vi "Demo_NIringData.vi"() -> ()   [LabVIEW 2021, in "RocketPlotDemo.lvlib"]
uses:
  Demo/RocketPlotDemo.lvlib
  TypeDefs/plot load data V2.ctl
  TypeDefs/plot properties V2.ctl
  TypeDefs/plot attributes V2.ctl
  TypeDefs/Plot scale axis properties.ctl
  TypeDefs/Plot general properties.ctl
  Classes/RocketPlotHandle/SubVIs/Init Options.ctl
  TypeDefs/TimeZone.ctl
  Classes/RocketPlotPanel/RocketPlotPanel.lvclass/RocketPlotPanel.ctl
  Demo/SubVIs/ring buffer data.ctl
  Classes/RocketPlotPanel/Read RocketPlotHandle.vi
  Classes/NIringPlotHandle/NIringPlotHandle.lvclass
  C:/Users/bjustice/Documents/GitHub/BluePlot/Source/Classes/RocketPlotHandle/RocketPlotHandle.lvclass
  Classes/RocketPlotPanel/RocketPlotPanel.lvclass
  C:/Program Files/National Instruments/LabVIEW 2021/vi.lib/IlluminatedG/IG OOPanel/OOPanel/Panel/Panel.lvclass
  Classes/RocketPlotHandle/Load PlotConfig.vi
  Classes/RocketPlotHandle/RocketPlotHandle.lvclass
  Classes/RocketPlotHandle/Get PlotConfig.vi
  <vilib>/National Instruments/Variant Ring Buffer/Ring Buffer.lvclass
  RocketPlot.lvlib
  <vilib>/IlluminatedG/IG OOPanel/OOPanel/Manager/Manager.lvclass
  C:/Users/bjustice/Documents/GitHub/BluePlot/Source/Classes/NIringPlotHandle/NIringPlotHandle.lvclass
  C:/Users/bjustice/Documents/GitHub/BluePlot/Source/Classes/RocketPlotPanel/RocketPlotPanel.lvclass
panel:
  in  "load config":bool
  in  "get config":bool
  out "time to plot":dbl
  out "Subscribed names":i32(listbox)
  in  "Plot config":T1={"plots"=[], "X-axis"={"Name Label.Text"="", "Style"=0, "Tick Colors:Minor Tick Color"=0, "Tick Colors:Tick Color"=0, "Marker Colors:Text Color"=0, "Grid Colors:Major Color"=0, "Grid Colors:Minor Color"=0, "Mapping Mode"=0, "Flipped"=FALSE, "Name Label.Visible"=FALSE, "Name Label.Text Colors:Text Color"=0, "Scale Fit"=0, "Range:Maximum"=0.0, "Range:Minimum"=0.0, "Offset and Multiplier:Multiplier"=0.0, "Offset and Multiplier:Offset"=0.0, "Name Label.Font:Size"=0, "Marker.Font:Size"=0, "Uniform Marker Spacing?"=TRUE, "Format String"=""}, "Y-axes"=[], "General"={"Title"="", "Time to Plot"=1800.0, "Title.Visible"=FALSE, "Sidebar.Visible"=FALSE, "Plot Area:Colors:BG Color"=0, "X Scale.Plot Name"="", "X Scale.Use Plot Name"=FALSE}} {"General"."Time to Plot" format="%<%M:%S>t"}
  # "Documentation and user guide:"
  # "https://github.com/justiceb/BluePlot/blob/main/README.md"
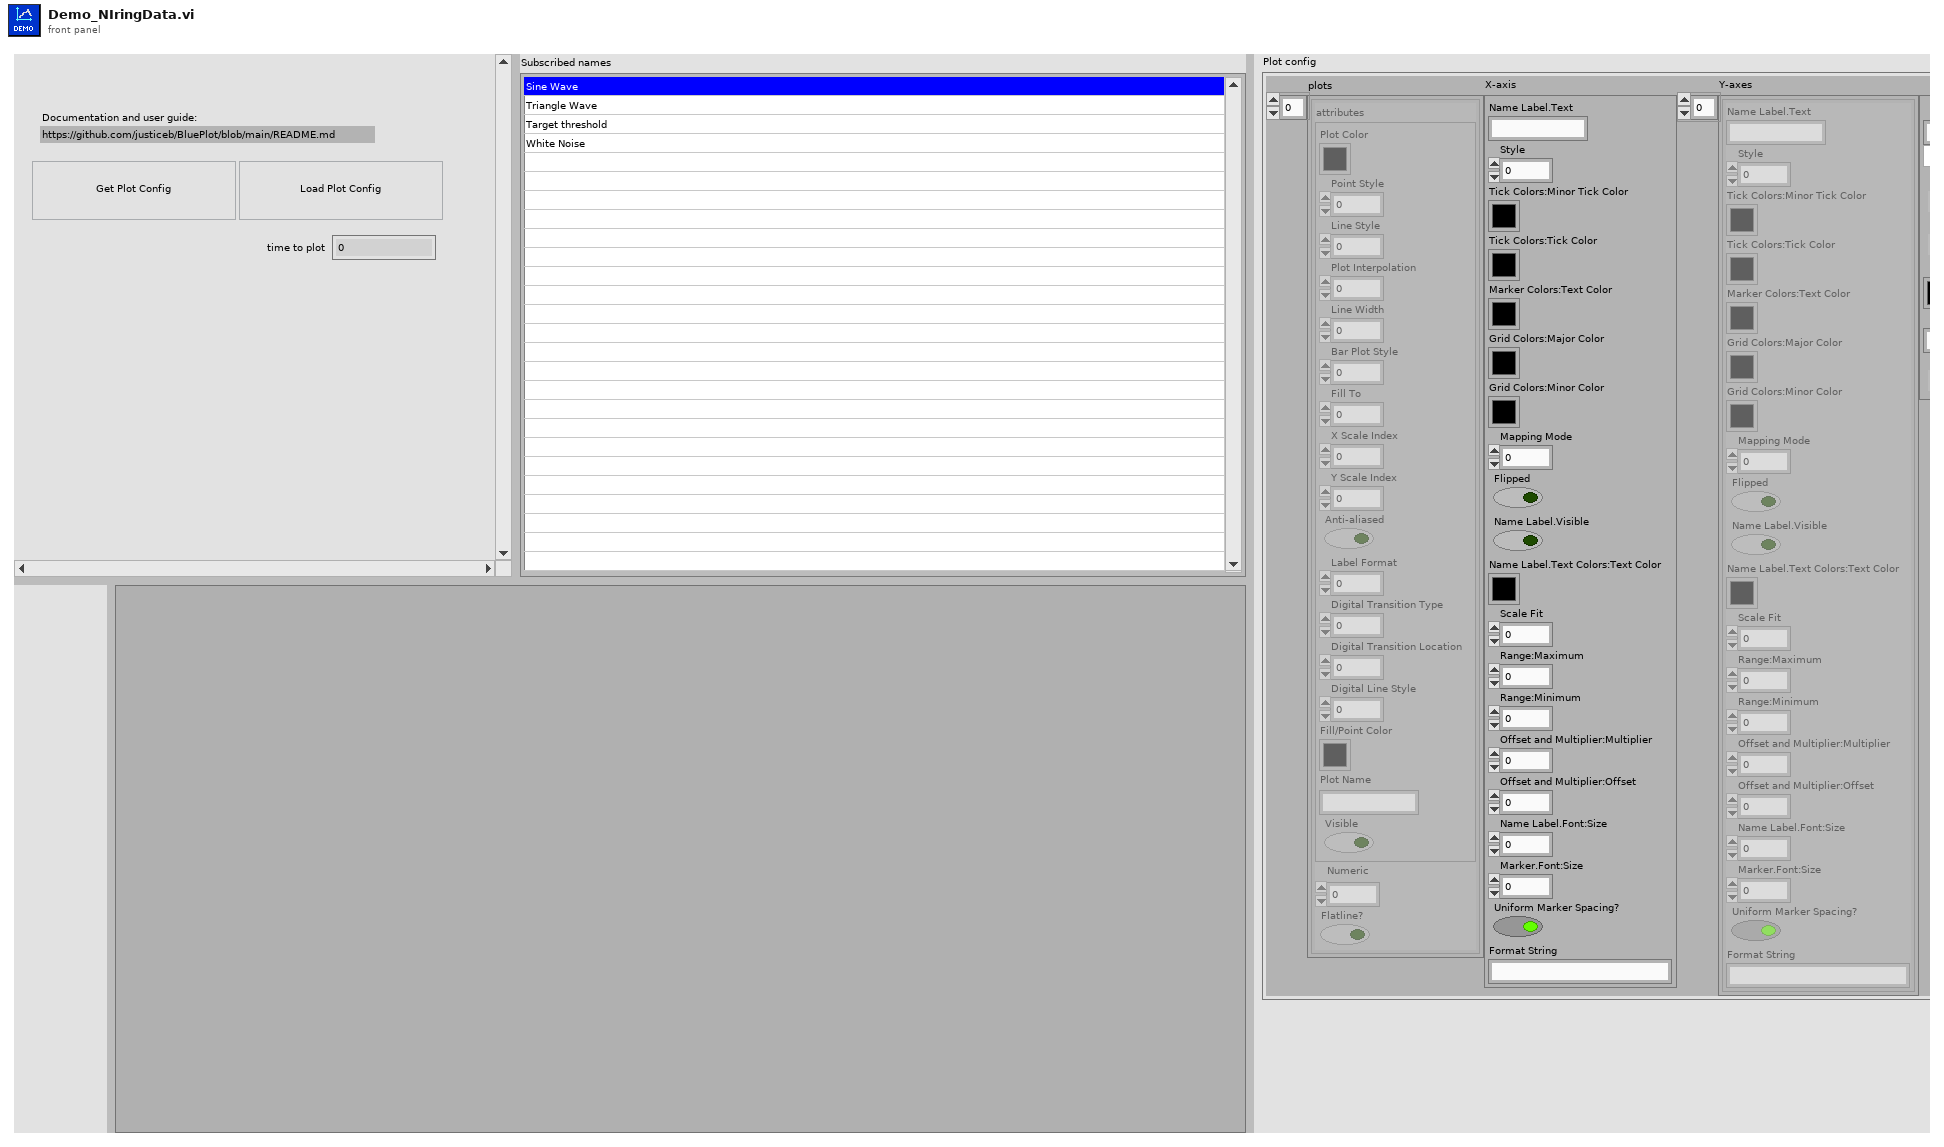
[diagram p1: front panel]
types:
  T1 = typedef "RocketPlot.lvlib/plot load data V2.ctl" = cluster{"plots":T2[], "X-axis":T4, "Y-axes":T4[], "General":T5}
  T2 = typedef "RocketPlot.lvlib/plot properties V2.ctl" = cluster{"attributes":T3, "Numeric":dbl, "Flatline?":bool}
  T3 = typedef "RocketPlot.lvlib/plot attributes V2.ctl" = cluster{"Plot Color":u32, "Point Style":u8, "Line Style":u8, "Plot Interpolation":u8, "Line Width":u8, "Bar Plot Style":u8, "Fill To":i16, "X Scale Index":u32, "Y Scale Index":u32, "Anti-aliased":bool, "Label Format":u8, "Digital Transition Type":u8, "Digital Transition Location":u8, "Digital Line Style":u8, "Fill/Point Color":u32, "Plot Name":string, "Visible":bool}
  T4 = typedef "RocketPlot.lvlib/Plot scale axis properties.ctl" = cluster{"Name Label.Text":string, "Style":u8, "Tick Colors:Minor Tick Color":u32, "Tick Colors:Tick Color":u32, "Marker Colors:Text Color":u32, "Grid Colors:Major Color":u32, "Grid Colors:Minor Color":u32, "Mapping Mode":u8, "Flipped":bool, "Name Label.Visible":bool, "Name Label.Text Colors:Text Color":u32, "Scale Fit":u8, "Range:Maximum":dbl, "Range:Minimum":dbl, "Offset and Multiplier:Multiplier":dbl, "Offset and Multiplier:Offset":dbl, "Name Label.Font:Size":u32, "Marker.Font:Size":u32, "Uniform Marker Spacing?":bool, "Format String":string}
  T5 = typedef "RocketPlot.lvlib/Plot general properties.ctl" = cluster{"Title":string, "Time to Plot":dbl, "Title.Visible":bool, "Sidebar.Visible":bool, "Plot Area:Colors:BG Color":u32, "X Scale.Plot Name":string, "X Scale.Use Plot Name":bool}
  T6 = typedef "RocketPlotHandle.lvclass/Init Options.ctl" = cluster{"UI visible?":bool, "Update rate (ms)":u32, "Sidebar.Visible":bool, "time to plot (init)":dbl, "time to plot (max)":dbl, "config file start path":path, "Title.Visible":bool, "Title":string, "TimeZone":T7}
  T7 = typedef "RocketPlot.lvlib/TimeZone.ctl" = enum16{"UTC", "Local"}
  T8 = typedef "RocketPlotDemo.lvlib/ring buffer data.ctl" = cluster{"timestamp":dbl, "value":dbl}
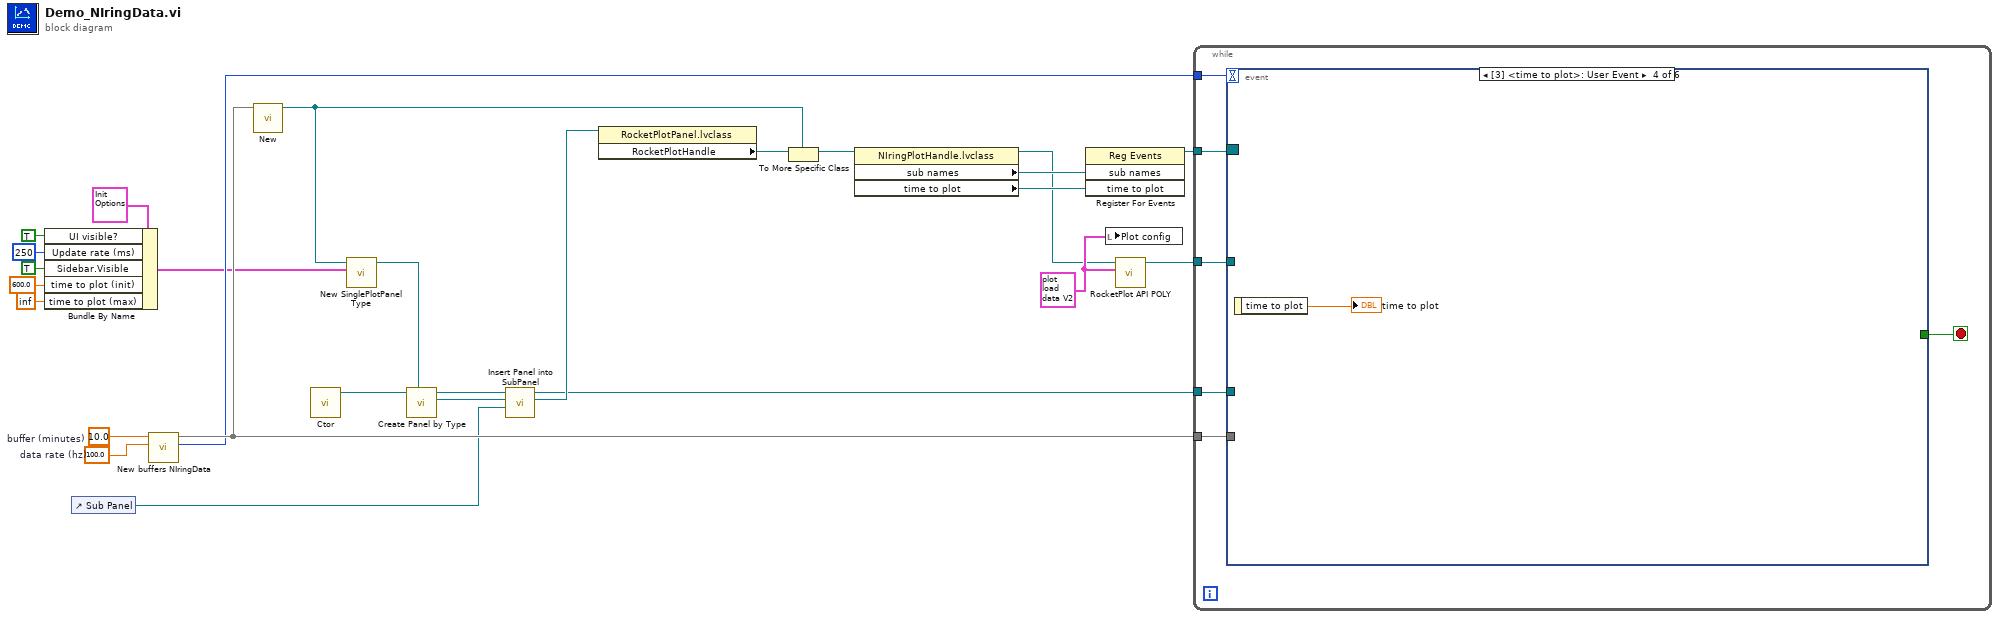
[diagram p0: block diagram]
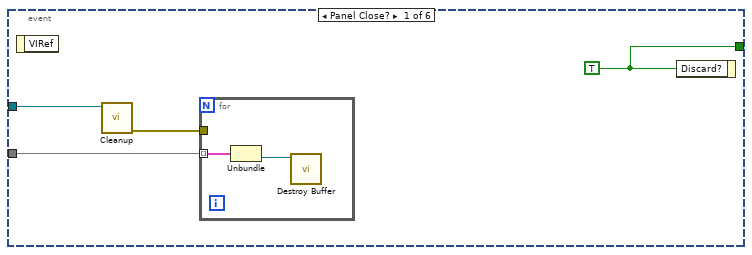
[diagram p2: hidden frame]
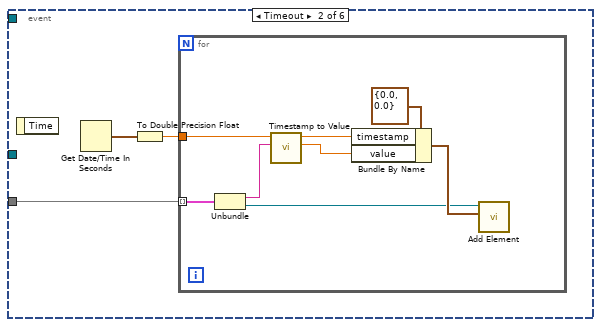
[diagram p3: hidden frame]
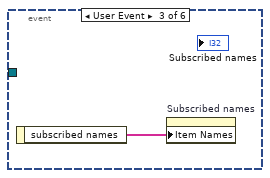
[diagram p4: hidden frame]
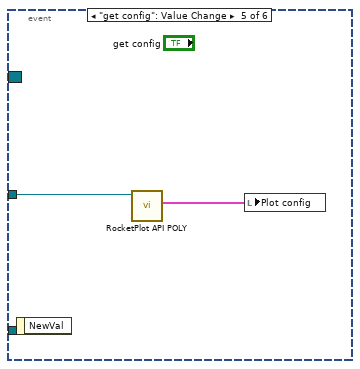
[diagram p5: hidden frame]
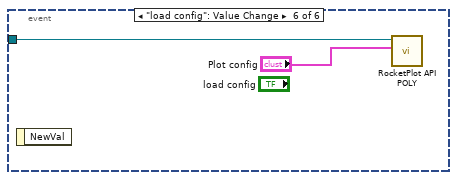
[diagram p6: hidden frame]
diagram:
  w21 = T1 {"plots"=[{"attributes"={"Plot Color"=16711680, "Point Style"=0, "Line Style"=0, "Plot Interpolation"=2, "Line Width"=0, "Bar Plot Style"=0, "Fill To"=-1, "X Scale Index"=0, "Y Scale Index"=0, "Anti-aliased"=FALSE, "Label Format"=3, "Digital Transition Type"=0, "Digital Transition Location"=2, "Digital Line Style"=1, "Fill/Point Color"=16711680, "Plot Name"="Sine Wave", "Visible"=TRUE}, "Numeric"=0.0, "Flatline?"=FALSE}, {"attributes"={"Plot Color"=4387583, "Point Style"=0, "Line Style"=0, "Plot Interpolation"=2, "Line Width"=0, "Bar Plot Style"=0, "Fill To"=-1, "X Scale Index"=0, "Y Scale Index"=1, "Anti-aliased"=FALSE, "Label Format"=3, "Digital Transition Type"=0, "Digital Transition Location"=2, "Digital Line Style"=1, "Fill/Point Color"=4387583, "Plot Name"="Triangle Wave", "Visible"=TRUE}, "Numeric"=0.0, "Flatline?"=FALSE}, {"attributes"={"Plot Color"=16722671, "Point Style"=0, "Line Style"=0, "Plot Interpolation"=2, "Line Width"=5, "Bar Plot Style"=0, "Fill To"=-1, "X Scale Index"=0, "Y Scale Index"=0, "Anti-aliased"=FALSE, "Label Format"=3, "Digital Transition Type"=0, "Digital Transition Location"=2, "Digital Line Style"=1, "Fill/Point Color"=16722671, "Plot Name"="Target threshold", "Visible"=TRUE}, "Numeric"=0.6, "Flatline?"=TRUE}, {"attributes"={"Plot Color"=16860, "Point Style"=0, "Line Style"=0, "Plot Interpolation"=2, "Line Width"=0, "Bar Plot Style"=0, "Fill To"=-1, "X Scale Index"=0, "Y Scale Index"=0, "Anti-aliased"=FALSE, "Label Format"=3, "Digital Transition Type"=0, "Digital Transition Location"=2, "Digital Line Style"=1, "Fill/Point Color"=16860, "Plot Name"="", "Visible"=TRUE}, "Numeric"=0.0, "Flatline?"=FALSE}], "X-axis"={"Name Label.Text"="Time (s)", "Style"=0, "Tick Colors:Minor Tick Color"=16777216, "Tick Colors:Tick Color"=3684408, "Marker Colors:Text Color"=16448250, "Grid Colors:Major Color"=3684408, "Grid Colors:Minor Color"=16777216, "Mapping Mode"=0, "Flipped"=FALSE, "Name Label.Visible"=TRUE, "Name Label.Text Colors:Text Color"=16448250, "Scale Fit"=2, "Range:Maximum"=3757348740.0, "Range:Minimum"=3757348080.0, "Offset and Multiplier:Multiplier"=1.0, "Offset and Multiplier:Offset"=0.0, "Name Label.Font:Size"=15, "Marker.Font:Size"=15, "Uniform Marker Spacing?"=TRUE, "Format String"="%<%H:%M:%S>T"}, "Y-axes"=[{"Name Label.Text"="Left Axis", "Style"=0, "Tick Colors:Minor Tick Color"=16777216, "Tick Colors:Tick Color"=3684408, "Marker Colors:Text Color"=16448250, "Grid Colors:Major Color"=3684408, "Grid Colors:Minor Color"=16777216, "Mapping Mode"=0, "Flipped"=FALSE, "Name Label.Visible"=FALSE, "Name Label.Text Colors:Text Color"=16448250, "Scale Fit"=2, "Range:Maximum"=1.0, "Range:Minimum"=-1.0, "Offset and Multiplier:Multiplier"=1.0, "Offset and Multiplier:Offset"=0.0, "Name Label.Font:Size"=15, "Marker.Font:Size"=15, "Uniform Marker Spacing?"=TRUE, "Format String"="%#_g"}, {"Name Label.Text"="Right Axis", "Style"=0, "Tick Colors:Minor Tick Color"=16777216, "Tick Colors:Tick Color"=3684408, "Marker Colors:Text Color"=16448250, "Grid Colors:Major Color"=3684408, "Grid Colors:Minor Color"=16777216, "Mapping Mode"=0, "Flipped"=FALSE, "Name Label.Visible"=FALSE, "Name Label.Text Colors:Text Color"=16448250, "Scale Fit"=0, "Range:Maximum"=1.0, "Range:Minimum"=-2.0, "Offset and Multiplier:Multiplier"=1.0, "Offset and Multiplier:Offset"=0.0, "Name Label.Font:Size"=15, "Marker.Font:Size"=15, "Uniform Marker Spacing?"=TRUE, "Format String"="%#_g"}], "General"={"Title"="Title", "Time to Plot"=600.0, "Title.Visible"=TRUE, "Sidebar.Visible"=TRUE, "Plot Area:Colors:BG Color"=0, "X Scale.Plot Name"="", "X Scale.Use Plot Name"=FALSE}} ("Plot config")
  w25 = 100.0  # data rate (hz)
  w26 = 10.0  # buffer (minutes)
  n1 = Bundle By Name(cluster=T6 {"UI visible?"=TRUE, "Update rate (ms)"=250, "Sidebar.Visible"=TRUE, "time to plot (init)"=600.0, "time to plot (max)"=inf, "config file start path"=path "", "Title.Visible"=TRUE, "Title"="Title", "TimeZone"=enum."Local"} ("Init options"), "UI visible?"=TRUE, "Update rate (ms)"=u32 250, "Sidebar.Visible"=TRUE ("visible sidebar?"), "time to plot (init)"=600.0, "time to plot (max)"=inf) -> (w14:T6)
  n2 = control-ref of="Sub Panel"() -> (w8:refnum<vi>)
  n3 = call "New buffers NIringData.vi"("data rate (hz)"=w25, "buffer (minutes)"=w26) -> ("period (ms)"=w23:i32, "ChannelMap"=w24:map{string, refnum<data-value>})  [unwired: 8 in]
  n4 = call "New.vi"("ChannelMap"=w24) -> ("plot handle"=w5:refnum<class "NIringPlotHandle.lvclass">)  [unwired: 9 in, 1 out]
  n5 = call <vilib>:"Ctor.vi"() -> ("Manager out"=w13:refnum<class "Manager.lvclass">)  [unwired: 10 in, 1 out]
  n6 = call "New SinglePlotPanel Type.vi"("Init options"=w14, "BluePlotHandle"=w5) -> ("SinglePlotPanel out"=w12:refnum<class "RocketPlotPanel.lvclass">)  [unwired: 8 in, 1 out]
  n7 = call <vilib>:"Create Panel by Type.vi"("Panel Type"=w12, "Manager in"=w13) -> ("Panel"=w10:refnum<class "RocketPlotPanel.lvclass">, "Manager out"=w11:refnum<class "Manager.lvclass">)  [unwired: 7 in, 1 out]
  n8 = call <vilib>:"Insert Panel into SubPanel.vi"("SubPanel"=w8, "Panel In"=w10, "Manager in"=w11) -> ("Panel"=w9:refnum<class "RocketPlotPanel.lvclass">, "Manager out"=w7:refnum<class "Manager.lvclass">)  [unwired: 6 in, 1 out]
  n9 = property class="RocketPlotPanel.lvclass"(reference=w9) -> ("RocketPlotHandle"=w6:refnum<class "RocketPlotHandle.lvclass">)  [unwired: 1 in, 2 out]
  n10 = To More Specific Class(target class=w5, reference=w6) -> (specific class reference=w4:refnum<class "NIringPlotHandle.lvclass">)  [unwired: 1 in, 1 out]
  n11 = property class="NIringPlotHandle.lvclass"(reference=w4) -> (reference out=w1:refnum<class "NIringPlotHandle.lvclass">, "sub names"=w3:refnum<user-event>, "time to plot"=w2:refnum<user-event>)  [unwired: 1 in, 1 out]
  n12 = register-events(w3, w2) -> (reference out=w27:refnum<event-registration>)  [unwired: 2 in, 1 out]
  n13 = local write "Plot config"(w21) -> ()
  n14 = call-poly "RocketPlot API POLY.vi"("Plot config"=w21, "BluePlotHandle in"=w1) -> ("BluePlotHandle out"=w22:refnum<class "NIringPlotHandle.lvclass">)  [unwired: 8 in, 1 out]
  n15 = while {
    tunnel: w22 -> [w33]
    tunnel: w27 -> [w31]
    tunnel: w24 -> [w30]
    tunnel: w23 -> [w29]
    tunnel: w7 -> [w28]
    stop <- w32 stop-if-true
    n16 = event shown="[3] <time to plot>: User Event" {
      selector: w31 -> [_ _ _ _ _ _]
      dyn-events: _ -> [_ _ _ _ _ _]
      timeout: w29 -> [_ _ _ _ _ _]
      tunnel: w33 -> [_ _ _ _ w54 w56]
      tunnel: [w36 _ _ _ _ _] -> w32
      tunnel: w30 -> [w37 w42 _ _ _ _]
      tunnel: w28 -> [w35 _ _ _ _ _]
      event Panel Close? {
        w36 = TRUE ("Discard?")
        n17 = event-data() -> ()  [unwired: 1 in, 1 out]
        n18 = call <vilib>:"Cleanup.vi"("Manager in"=w35) -> ("error out"=w34:errorcluster)  [unwired: 8 in, 2 out]
        n19 = for {
          tunnel: w34 -> [_]
          tunnel: w37 -> [w39] mode=indexing
          n20 = Unbundle(w39) -> ("Ring Buffer"=w38:refnum<data-value>)  [unwired: 1 out]
          n21 = call <vilib>:"Destroy Buffer.vi"("Ring Buffer Reference"=w38) -> ()  [unwired: 9 in, 2 out]
        }
        n22 = event-data("Discard?"=w36) -> ()  [unwired: 1 in, 1 out]
      }
      event Timeout {
        n23 = event-data() -> ()  [unwired: 1 in, 1 out]
        n24 = Get Date/Time In Seconds() -> (seconds since 1Jan1904=w41:timestamp)
        n25 = To Double Precision Float(number=w41) -> (double precision float=w40:dbl)
        n26 = for {
          tunnel: w42 -> [w45] mode=indexing
          tunnel: w40 -> [w50]
          n27 = Unbundle(w45) -> ("name"=w44:string, "Ring Buffer"=w43:refnum<data-value>)
          n28 = call "Timestamp to Value.vi"("name"=w44, "timestamp"=w50) -> ("value"=w47:dbl, "timestamp (dup)"=w48:dbl)  [unwired: 8 in]
          n29 = Bundle By Name(cluster=T8 {"timestamp"=0.0, "value"=0.0} ("Cluster"), "timestamp"=w48, "value"=w47) -> (w46:T8)
          n30 = call <vilib>:"Add Element.vi"("Variant"=w46, "Ring Buffer Reference"=w43) -> ()  [unwired: 8 in, 2 out]
        }
      }
      event User Event {
        n31 = event-data() -> ("subscribed names"=w51:string[])  [unwired: 1 in]
        n32 = property on="Subscribed names" class="LstBox (strict)"("Item Names"=w51) -> ()  [unwired: 2 in, 2 out]
      }
      event User Event {
        n33 = event-data() -> ("time to plot"=→"time to plot":dbl)  [unwired: 1 in]
      }
      event "get config": Value Change {
        n34 = event-data() -> ()  [unwired: 1 in, 1 out]
        n35 = call-poly "RocketPlot API POLY.vi"("BluePlotHandle in"=w54) -> ("Plot config"=w53:T1)  [unwired: 8 in, 2 out]
        n36 = local write "Plot config"(w53) -> ()
      }
      event "load config": Value Change {
        n37 = event-data() -> ()  [unwired: 1 in, 1 out]
        n38 = call-poly "RocketPlot API POLY.vi"("Plot config"="Plot config", "BluePlotHandle in"=w56) -> ()  [unwired: 8 in, 2 out]
      }
    }
  }
